vi "ConvertToSpreadsheet.vi"(10 "Kolonner":i32=4, 11 "Array in":dbl[](array[numeric])) -> (3 "Array out":string[][](array[string]))   [LabVIEW 2015]
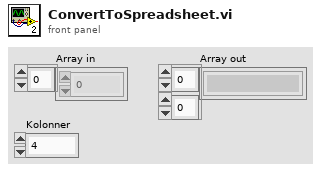
[diagram p1: front panel]
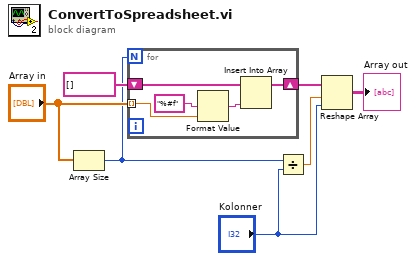
[diagram p0: block diagram]
diagram:
  n1 = Array Size(array="Array in") -> (size(s)=w4:i32)
  n2 = for {
    N: w4 -> [_]
    tunnel: "Array in" -> [w9] mode=indexing
    shift-right: [w11] -> w5
    shift-left: string[] [] ("Array") -> [w12]
    n3 = Format Value(format string="%#f", value (0)=w9) -> (output string=w8:string)  [unwired: 1 in]
    n4 = Insert Into Array(array=w12, new element=w8) -> (w11:string[])  [unwired: 1 in]
  }
  n5 = Divide(x=w4, y="Kolonner") -> (x/y=w2:dbl)
  n6 = Reshape Array(w5, w2, "Kolonner") -> (→"Array out":string[][])
